vi "signal1.vi"() -> ()   [LabVIEW 2021]
uses:
  <vilib>/Waveform/WDTFileIO.llb/Export Waveforms To Spreadsheet File (1D).vi
  <vilib>/measure/NI_MABase.lvlib
panel:
  out "Waveform Graph":waveform(dbl)[](graph)
  in  "Phase":dbl
  in  "Amplitude":dbl
  in  "Frequency":dbl
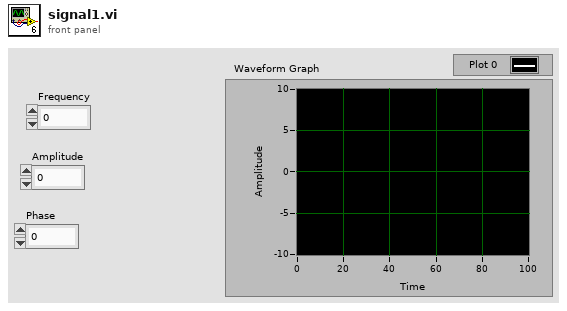
[diagram p1: front panel]
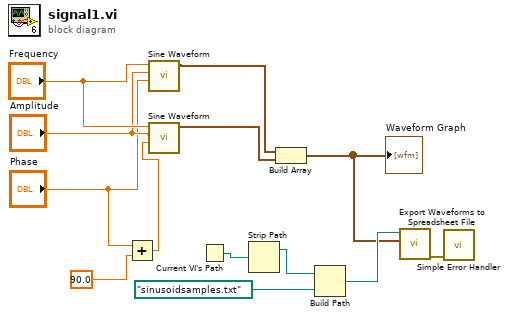
[diagram p0: block diagram]
diagram:
  n1 = Add(x="Phase", y=90.0) -> (x+y=w9:dbl)
  n2 = call <vilib>:"Sine Waveform.vi"("phase"="Phase", "amplitude"="Amplitude", "frequency"="Frequency") -> ("signal out"=w8:waveform(dbl))  [unwired: 7 in, 1 out]
  n3 = call <vilib>:"Sine Waveform.vi"("phase"=w9, "amplitude"="Amplitude", "frequency"="Frequency") -> ("signal out"=w7:waveform(dbl))  [unwired: 7 in, 1 out]
  n4 = Current VI's Path() -> (path=w4:path)
  n5 = Strip Path(path=w4) -> (stripped path=w6:path)  [unwired: 1 out]
  n6 = Build Array(w8, w7) -> (w1:waveform(dbl)[])
  "Waveform Graph" <- w1
  n7 = Build Path(base path=w6, name or relative path=path "sinusoidsamples.txt") -> (appended path=w2:path)
  n8 = call-poly <vilib>:"Export Waveforms to Spreadsheet File.vi"("waveforms"=w1, "file path (dialog if empty)"=w2) -> ("error out"=w3:errorcluster)  [unwired: 8 in, 1 out]
  n9 = call <vilib>:"Simple Error Handler.vi"("error in (no error)"=w3) -> ()  [unwired: 4 in, 5 out]
